vi "Process.vi"(8 "error in":errorcluster, 11 "Inst.RP100":refnum<class "Inst.RP100.lvclass">) -> (0 "error out":errorcluster, 3 "Inst.RP100 out":refnum<class "Inst.RP100.lvclass">)   [LabVIEW 2019, in "Inst.RP100.lvlib" / "Inst.RP100.lvclass"]
doc: "---------------------------------------------------------------\nJKI State Machine Objects™\nhttp://jki.net/state-machine-objects/\nCopyright (C) 2005-2015, JKI <info@jki.net>\nALL RIGHTS RESERVED"
uses:
  Inst.RP100.lvclass
  <userlib>/LevyLab/Instrument Framework/Instrument/Instrument.lvclass
  <userlib>/LevyLab/RemoteControl/RemoteControl/Typedefs/Message--Cluster.ctl
  <userlib>/LevyLab/RemoteControl/RemoteControl/RemoteControl.lvclass
  Typedefs/PrivateEvents--Inst.RP100.MessageToProcess.ctl
  C:/Program Files (x86)/National Instruments/LabVIEW 2019/user.lib/LevyLab/Instrument Framework/Instrument Types/Strain/Instrument.Strain.lvclass
  C:/Program Files (x86)/National Instruments/LabVIEW 2019/user.lib/LevyLab/Instrument Framework/Instrument/Instrument.lvclass
  C:/Program Files (x86)/National Instruments/LabVIEW 2019/vi.lib/JKI/JKI SMO/SMO/SMO.lvclass
  <userlib>/LevyLab/Debug/Debug.lvlib
  <vilib>/JKI/JKI SMO/SMO/SMO.lvclass
  <userlib>/LevyLab/Instrument Framework/Instrument Types/Strain/Instrument.Strain.lvclass
panel:
  out "Status":string
  out "State History":string
  # "Inst.RP100"
  # "Inst.RP100"
  # "For instructions on how to use the JKI State Machine Objects, examples and video tutorials, visit:\nhttp://jki.net/state-machine-objects/\n\nJKI State Machine Objects™\nhttp://jki.net/state-machine-objects/\nCopyright (C) 2005-2015, JKI <info@jki.net>\nALL RIGHTS RESERVED"
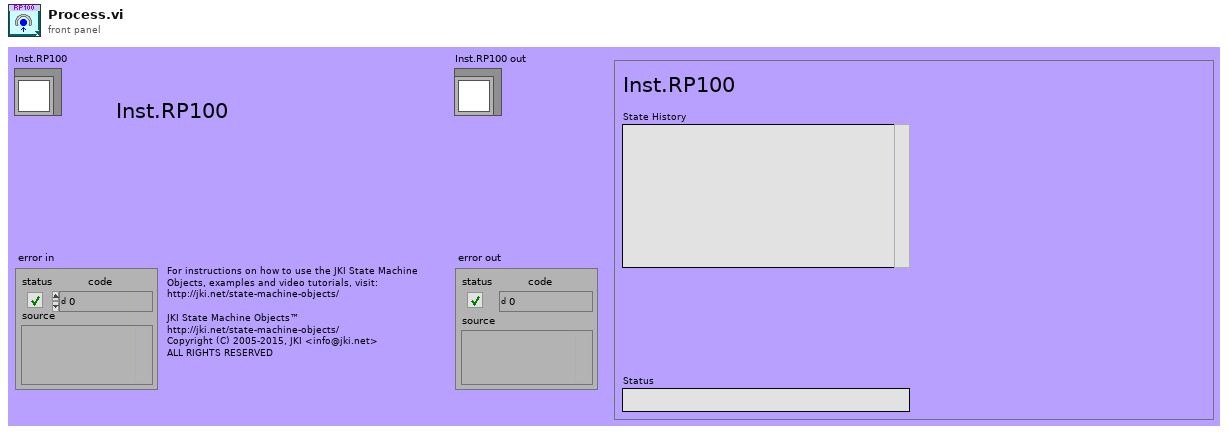
[diagram p1: front panel]
types:
  T1 = enum32{"invalid app kind", "Development System", "Run Time System", "Student Edition", "Embedded LabVIEW", "Evaluation", "Custom"}
  T2 = enum32{"Invalid", "Standard", "Closed", "Hidden", "Minimized", "Maximized"}
  T3 = typedef "RemoteControl.lvlib/RemoteControl.lvclass/Message--Cluster.ctl" = cluster{"Command":string, "Data":variant, "ID":string, "error":errorcluster}
  T4 = typedef "Inst.RP100.lvlib/Inst.RP100.lvclass/PrivateEvents--Inst.RP100.MessageToProcess.ctl" = cluster{"Message":T3}
  T5 = cluster{"Core":cluster{"Current VI Reference":refnum<vi>, "Close Panel on Exit?":bool, "Last Error":cluster{"error":errorcluster, "previous state":string, "remaining states":string}, "Shutdown?":bool}, "SMO":refnum<class "Inst.RP100.lvclass">, "Running Step":i32, "sequence":string[], "MessageToProcess":T4}
  T6 = cluster{"Current VI Reference":refnum<vi>, "Close Panel on Exit?":bool, "Last Error":cluster{"error":errorcluster, "previous state":string, "remaining states":string}, "Shutdown?":bool}
  T7 = typedef "Debug.lvlib/Attribute.Debug.lvclass/DebugBehavior.ctl" = enum16{"Normal", "Debug"}
  T8 = typedef "SMO.lvclass/Protected Events.ctl" = cluster{"StopProcesses":refnum<user-event>, "AbortProcesses":refnum<user-event>, "Config Changed":refnum<user-event>, "Dependency":refnum<user-event>}
  T9 = typedef "Inst.RP100.lvlib/Inst.RP100.lvclass/Inst.RP100.getAll--Cluster.ctl" = cluster{"OutputStateCh1":string, "OutputStateCh2":string, "LevelCh1":dbl, "LevelCh2":dbl, "SlewCh1":dbl, "SlewCh2":dbl, "MeasuredVCh1":dbl, "MeasuredVCh2":dbl, "MeasuredICh1":dbl, "MeasuredICh2":dbl}
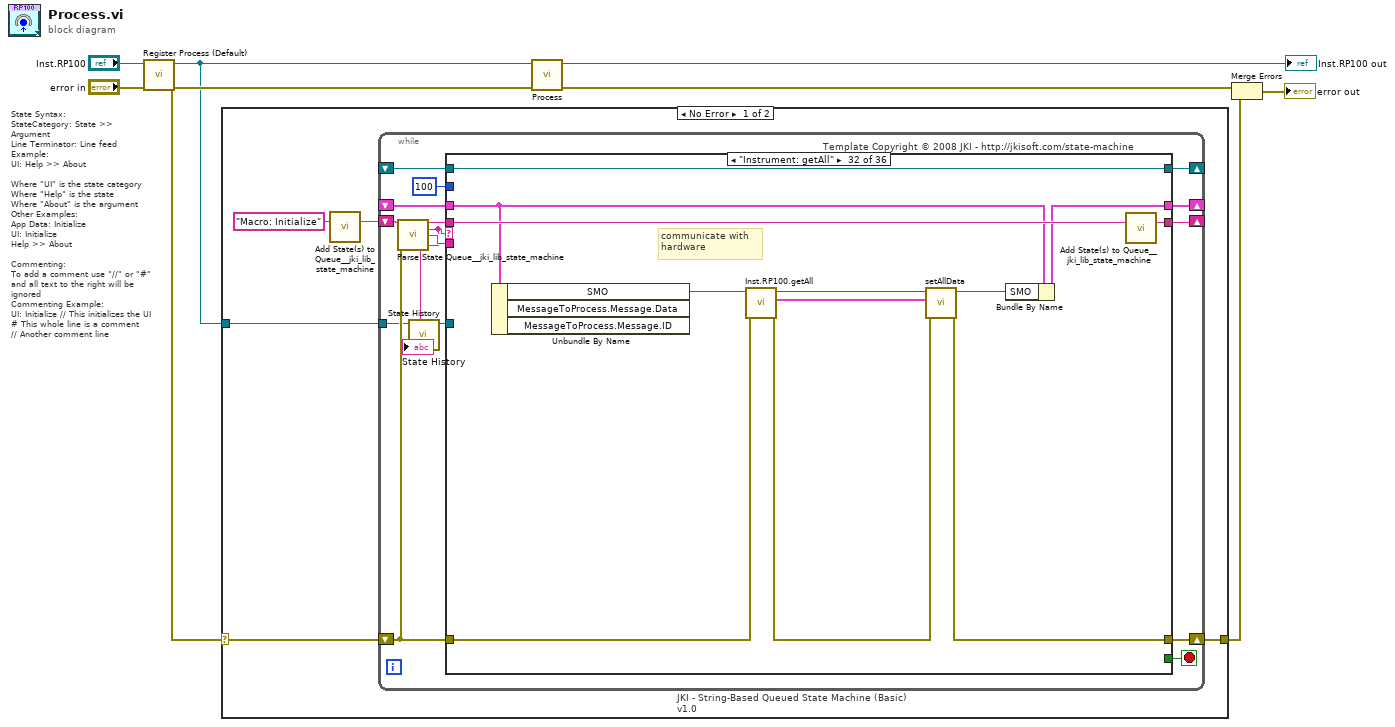
[diagram p0: block diagram]
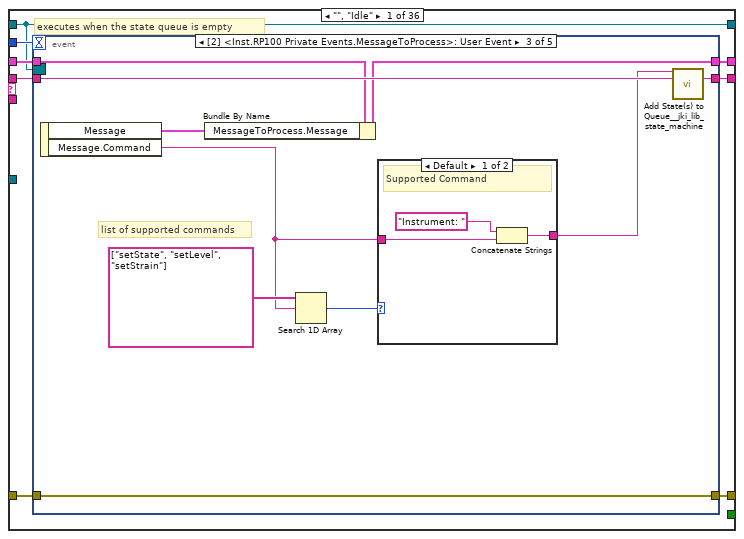
[diagram p2: hidden frame]
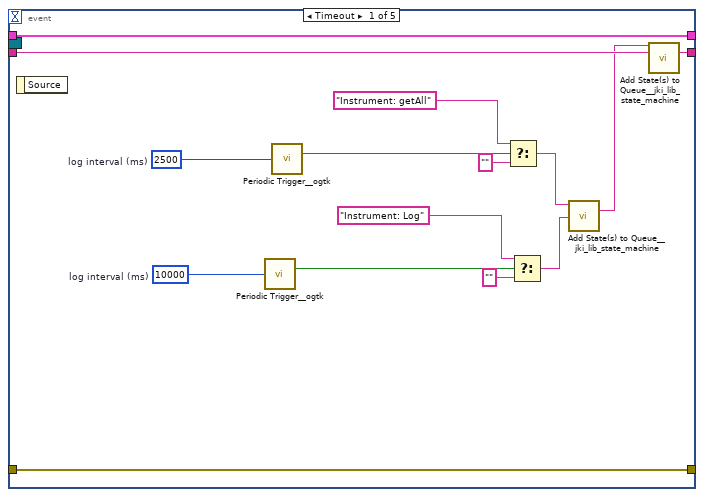
[diagram p3: hidden frame]
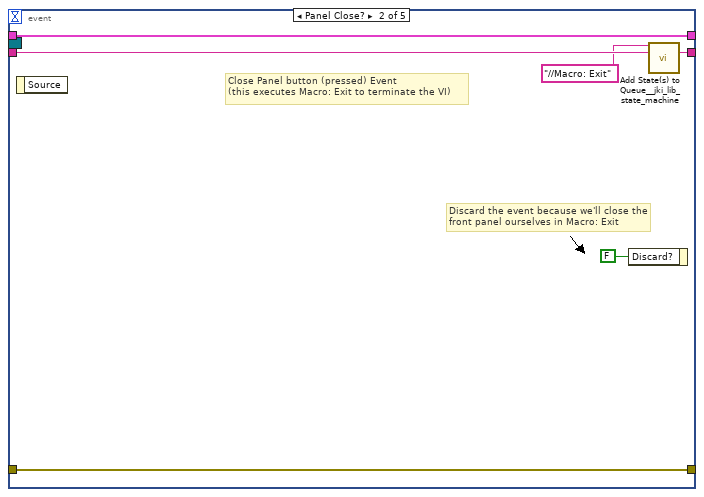
[diagram p4: hidden frame]
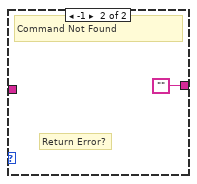
[diagram p5: hidden frame]
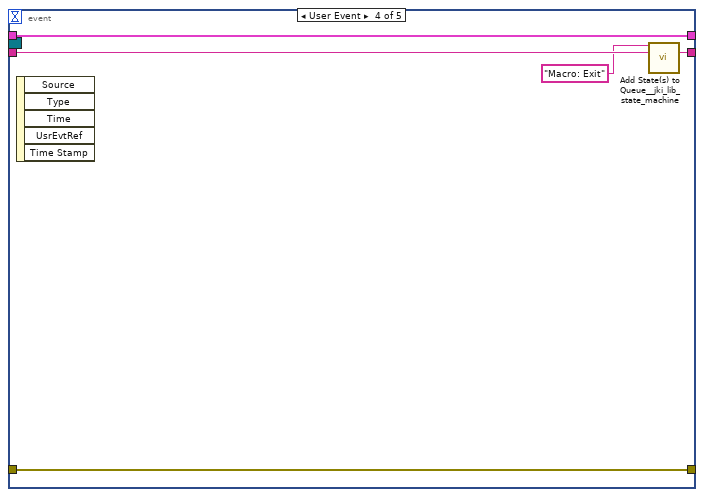
[diagram p6: hidden frame]
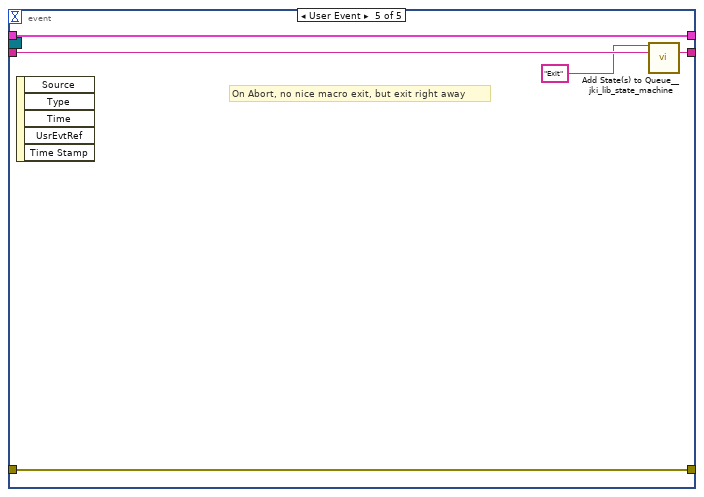
[diagram p7: hidden frame]
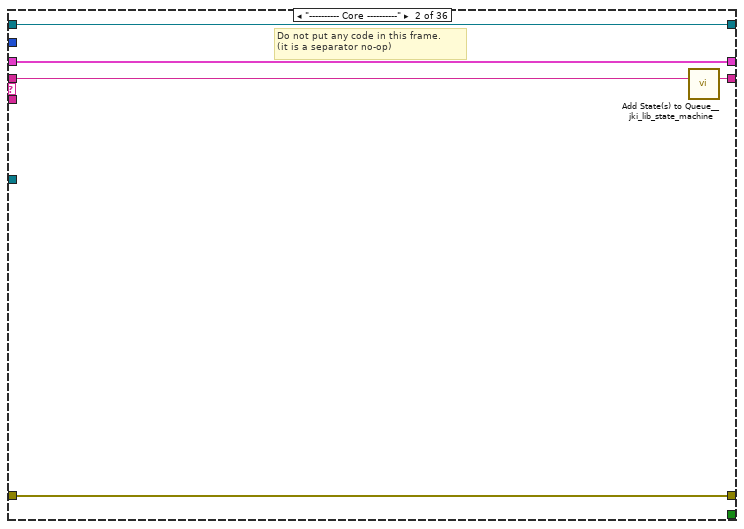
[diagram p8: hidden frame]
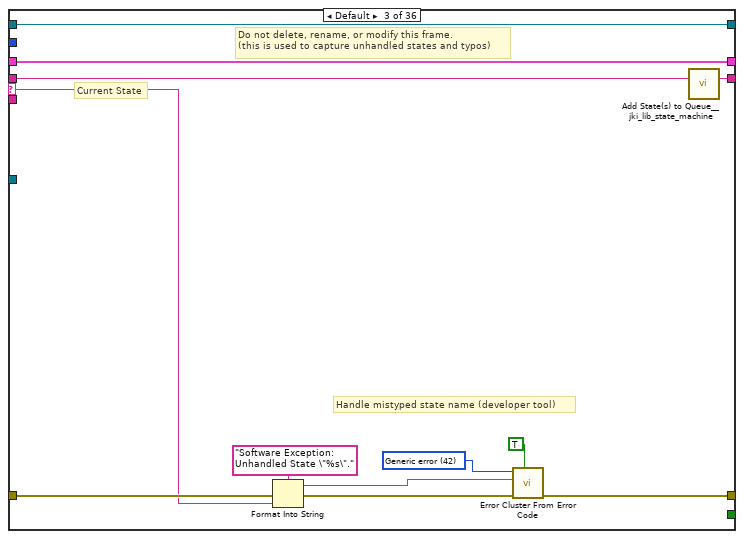
[diagram p9: hidden frame]
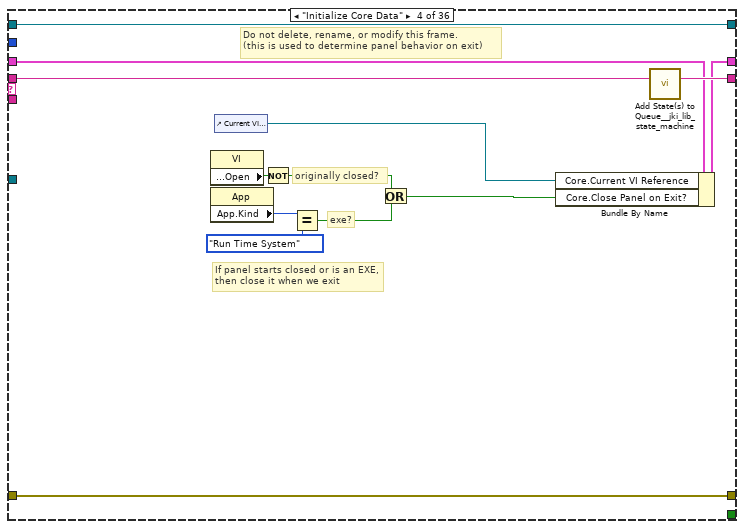
[diagram p10: hidden frame]
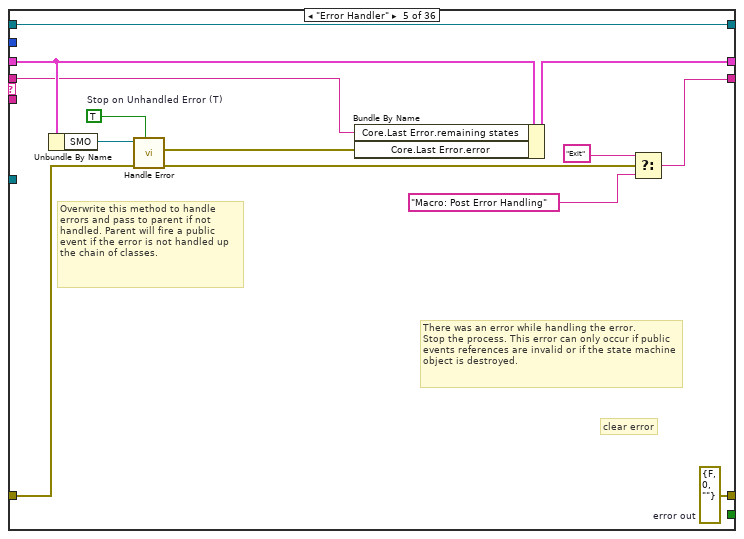
[diagram p11: hidden frame]
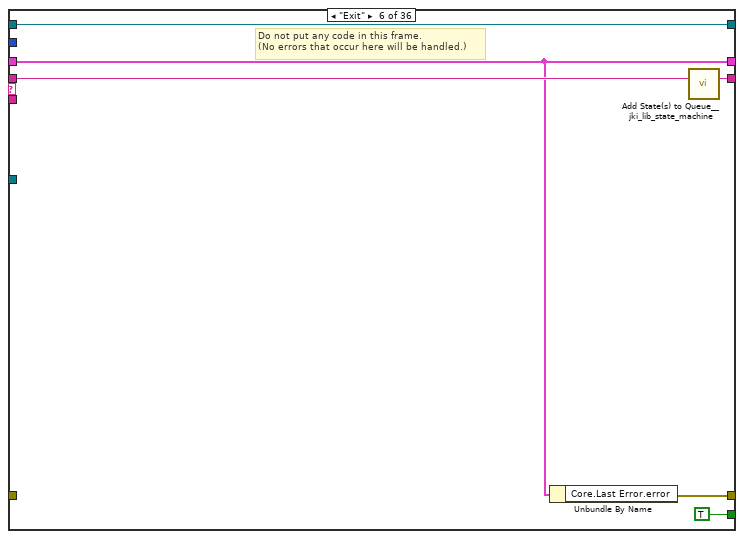
[diagram p12: hidden frame]
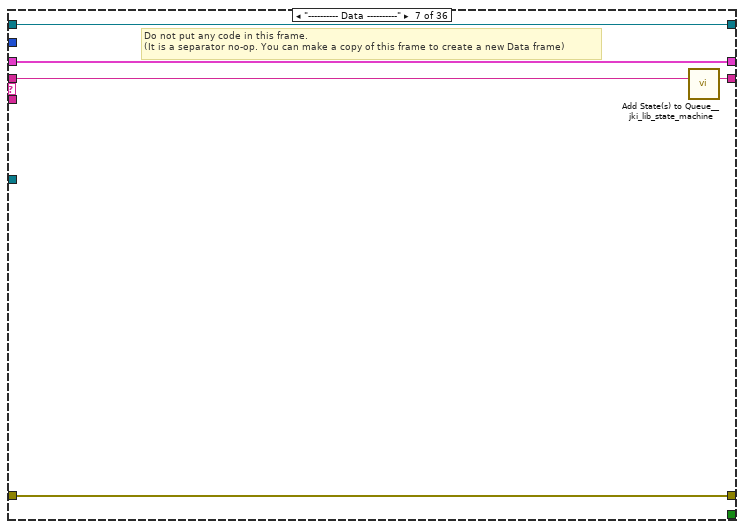
[diagram p13: hidden frame]
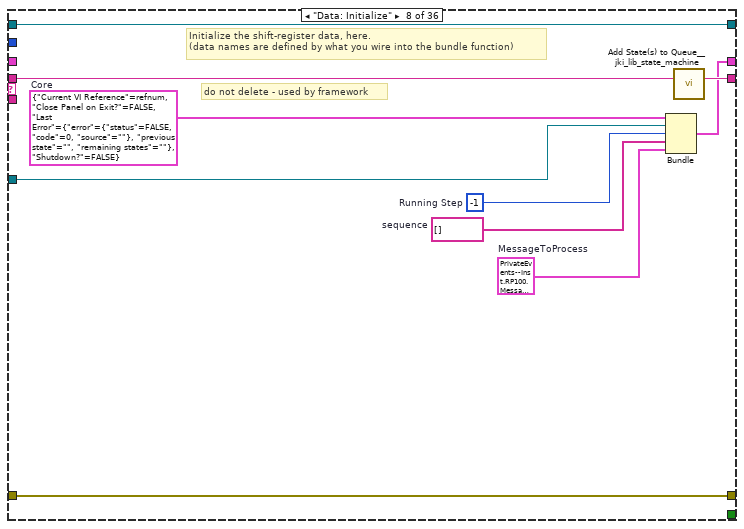
[diagram p14: hidden frame]
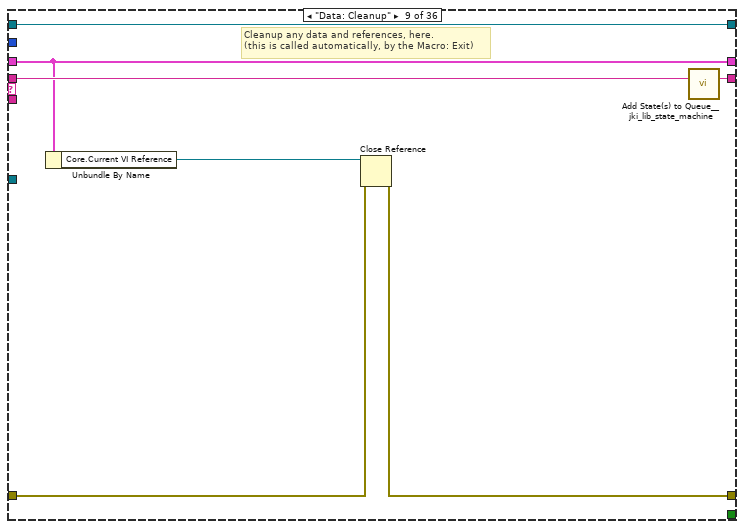
[diagram p15: hidden frame]
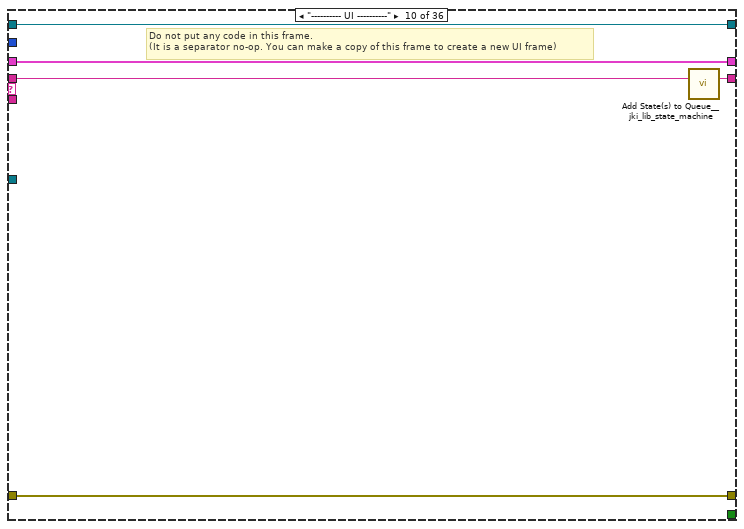
[diagram p16: hidden frame]
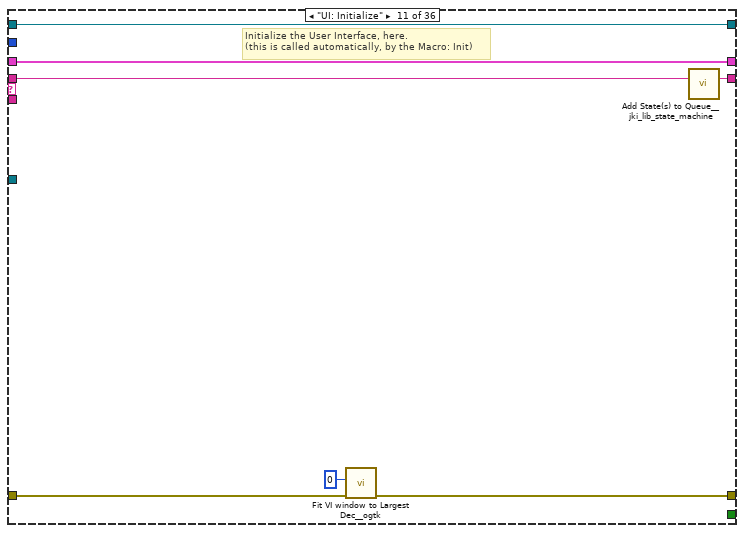
[diagram p17: hidden frame]
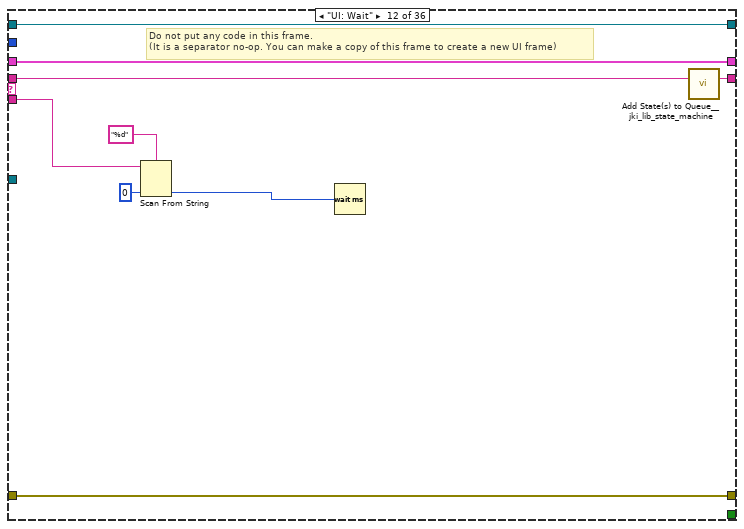
[diagram p18: hidden frame]
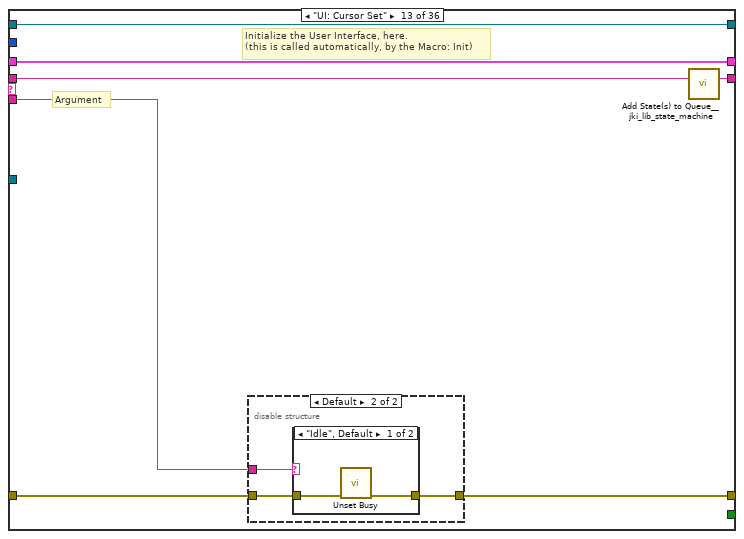
[diagram p19: hidden frame]
diagram:
  # "State Syntax:\nStateCategory: State >> Argument\nLine Terminator: Line feed\nExample:\nUI: Help >> About\n\nWhere \"UI\" is the state category\nWhere \"Help\" is the state\nWhere \"About\" is the argument\nOther Examples:\nApp Data: Initialize\nUI: Initialize\nHelp >> About\n\nCommenting:\nTo add a comment use \"//\" or \"#\" and all text to the right will be ignored\nCommenting Example:\nUI: Initialize // This initializes the UI\n# This whole line is a comment\n// Another comment line"
  n1 = call <vilib>:"Register Process (Default).vi"("error in (no error)"="error in", "SMO"="Inst.RP100") -> ("error out"=w5:errorcluster, "SelfRef"=w4:refnum<class "Inst.RP100.lvclass">)  [unwired: 8 in]
  n2 = case shown="No Error" w5 {
    selector: w5 -> [w10 w459]
    tunnel: w4 -> [w11 _]
    tunnel: [w9 w459] -> w1
    frame No Error {
      n3 = call <vilib>:"Add State(s) to Queue__jki_lib_state_machine.vi"("State(s) in (\"\")"="Macro: Initialize") -> ("States Out"=w13:string)  [unwired: 14 in]
      n4 = while "JKI - String-Based Queued State Machine (Basic) v1.0" {
        shift-right: [w23] -> _
        shift-left: _ -> [w22]
        shift-right: [w26] -> w9
        shift-left: w10 -> [w20]
        shift-right: [w25] -> _
        shift-left: w13 -> [w27]
        tunnel: w11 -> [w14]
        shift-right: [w19] -> _
        shift-left: _ -> [w18]
        stop <- w24 stop-if-true
        # "Template Copyright © 2008 JKI - http://jkisoft.com/state-machine"
        n5 = call <vilib>:"Parse State Queue__jki_lib_state_machine.vi"("State Queue"=w27, "Error In (no error)"=w20) -> ("Remaining States"=w29:string, "Current State"=w17:string, "Arguments"=w28:string)  [unwired: 11 in]
        n6 = call <userlib>:"State History.vi"("Current State"=w17, "SMO"=w14) -> ("SMO"=w15:refnum<class "Inst.RP100.lvclass">, "History"=→"State History":string)  [unwired: 8 in]
        n7 = case shown="\"Instrument: getAll\"" w17 {
          selector: w17 -> [_ _ w89 _ _ _ _ _ _ _ _ _ _ _ _ _ _ _ _ _ _ _ _ _ _ _ _ _ _ _ _ _ _ _ _ _]
          tunnel: w29 -> [w37 w87 w93 w112 w117 w131 w136 w146 w153 w158 w165 w174 w181 w197 w229 w238 w253 w270 w291 w308 w313 w324 w329 w342 w348 w355 w364 w373 w383 w393 w403 w415 w428 w433 w439 w458]
          tunnel: w28 -> [_ _ _ _ _ _ _ _ _ _ _ w166 w175 w191 _ _ _ _ _ _ _ _ _ _ _ _ _ _ _ _ _ _ _ _ w434 w442]
          tunnel: w22 -> [w35 w84 w91 w103 w121 w127 w133 _ w147 w155 w163 w171 w179 w193 w226 w235 w242 w260 w281 w292 w310 w321 w326 w335 w346 w350 w360 w369 w379 w389 w399 w411 w424 w429 w435 w448]
          tunnel: [w34 w85 w95 w109 w122 w126 w134 w138 w149 w156 w160 w172 w176 w194 w227 w230 w240 w268 w289 w295 w311 w315 w327 w338 w344 w352 w357 w366 w375 w385 w395 w404 w418 w430 w436 w450] -> w26
          tunnel: w20 -> [w33 w85 w94 w109 w123 _ w134 w138 w150 w156 w159 w172 w177 w195 w227 w230 w239 w268 w289 w295 w311 w316 w327 w332 w344 w352 w356 w365 w376 w386 w396 w409 w419 w430 w436 w444]
          tunnel: [w36 w86 w92 w111 w113 w130 w135 w145 w152 w157 w164 w173 w180 w196 w228 w237 w252 w269 w290 w307 w312 w323 w328 w341 w347 w354 w363 w372 w382 w392 w402 w414 w427 w432 w438 w457] -> w25
          tunnel: [_ _ _ _ _ TRUE _ _ _ _ _ _ _ _ _ _ _ _ _ _ _ _ _ _ _ _ _ _ _ _ _ _ _ _ _ _] -> w24
          tunnel: [w32 w84 w91 w110 w120 w127 w133 w144 w147 w155 w163 w171 w179 w193 w226 w235 w243 w261 w282 w293 w310 w321 w326 w335 w346 w351 w361 w370 w380 w390 w400 w412 w425 w429 w435 w447] -> w23
          tunnel: 100 ("Timeout") -> [w31 _ _ _ _ _ _ _ _ _ _ _ _ _ _ _ _ _ _ _ _ _ _ _ _ _ _ _ _ _ _ _ _ _ _ _]
          tunnel: w15 -> [_ _ _ _ _ _ _ w139 _ _ _ _ _ _ _ _ _ _ _ _ _ _ _ _ _ _ _ _ _ _ _ _ _ _ _ _]
          tunnel: [w30 w83 w88 w100 w125 w128 w132 w143 w148 w154 w162 w170 w178 w190 w225 w236 w251 w267 w288 w302 w309 w322 w325 w340 w345 w353 w362 w371 w381 w391 w401 w413 w426 w431 w437 w456] -> w19
          tunnel: w18 -> [w30 w83 w88 w100 w125 w128 w132 w143 w148 w154 w162 w170 w178 w190 w225 w236 w251 w267 w288 w302 w309 w322 w325 _ w345 w353 w362 w371 w381 w391 w401 w413 w426 w431 w437 w456]
          frame "", "Idle" {
            # "executes when the state queue is empty"
            n8 = event shown="[2] <Inst.RP100 Private Events.MessageToProcess>: User Event" {
              selector: w30 -> [_ _ _ _ _]
              dyn-events: _ -> [_ _ _ _ _]
              timeout: w31 -> [_ _ _ _ _]
              tunnel: w37 -> [w52 w58 w68 w77 w82]
              tunnel: [w51 w57 w67 w76 w81] -> w36
              tunnel: w35 -> [w49 w55 w60 w74 w79]
              tunnel: [w50 w56 w66 w75 w80] -> w34
              tunnel: w33 -> [w50 w56 w66 w75 w80]
              tunnel: [w49 w55 w61 w74 w79] -> w32
              event Timeout {
                w42 = u32 10000  # log interval (ms)
                w46 = u32 2500  # log interval (ms)
                n9 = event-data() -> ()  [unwired: 1 in, 1 out]
                n10 = call <userlib>:"Periodic Trigger__ogtk.vi"("time (ms)"=w42) -> ("Triggered"=w41:bool)  [unwired: 12 in, 2 out]
                n11 = call <userlib>:"Periodic Trigger__ogtk.vi"("time (ms)"=w46) -> ("Triggered"=w48:bool)  [unwired: 12 in, 2 out]
                n12 = Select(t="Instrument: getAll", s=w48, f="") -> (s? t:f=w39:string)
                n13 = Select(t="Instrument: Log", s=w41, f="") -> (s? t:f=w40:string)
                n14 = call <vilib>:"Add State(s) to Queue__jki_lib_state_machine.vi"("State(s) in Front (\"\")"=w39, "State(s) at Back (\"\")"=w40) -> ("States Out"=w38:string)  [unwired: 13 in]
                n15 = call <vilib>:"Add State(s) to Queue__jki_lib_state_machine.vi"("State(s) in Front (\"\")"=w38, "State(s) in (\"\")"=w52) -> ("States Out"=w51:string)  [unwired: 13 in]
              }
              event Panel Close? {
                # "Discard the event because we'll close the front panel ourselves in Macro: Exit"
                # "Close Panel button (pressed) Event\n(this executes Macro: Exit to terminate the VI)"
                n16 = event-data() -> ()  [unwired: 1 in, 1 out]
                n17 = event-data("Discard?"=FALSE) -> ()  [unwired: 1 in, 1 out]
                n18 = call <vilib>:"Add State(s) to Queue__jki_lib_state_machine.vi"("State(s) in Front (\"\")"="//Macro: Exit", "State(s) in (\"\")"=w58) -> ("States Out"=w57:string)  [unwired: 13 in]
              }
              event User Event {
                # "list of supported commands"
                n19 = event-data() -> ("Message"=w59:T3, "Message.Command"=w62:string)  [unwired: 1 in]
                n20 = Bundle By Name(cluster=w60, "MessageToProcess.Message"=w59) -> (w61:T5)
                n21 = Search 1D Array(1D array=string[] ["setState", "setLevel", "setStrain"], element=w62) -> (index of element=w65:i32)  [unwired: 1 in]
                n22 = case shown="Default" w65 {
                  tunnel: [w71 "" ("Empty String Constant")] -> w63
                  tunnel: w62 -> [w70 _]
                  frame Default {
                    # "Supported Command"
                    n23 = Concatenate Strings("Instrument: ", w70) -> (w71:string)
                  }
                  frame -1 {
                    # "Return Error?"
                    # "Command Not Found"
                  }
                }
                n24 = call <vilib>:"Add State(s) to Queue__jki_lib_state_machine.vi"("State(s) in Front (\"\")"=w63, "State(s) in (\"\")"=w68) -> ("States Out"=w67:string)  [unwired: 13 in]
              }
              event User Event {
                n25 = event-data() -> ()  [unwired: 1 in, 5 out]
                n26 = call <vilib>:"Add State(s) to Queue__jki_lib_state_machine.vi"("State(s) in Front (\"\")"="Macro: Exit", "State(s) in (\"\")"=w77) -> ("States Out"=w76:string)  [unwired: 13 in]
              }
              event User Event {
                # "On Abort, no nice macro exit, but exit right away"
                n27 = event-data() -> ()  [unwired: 1 in, 5 out]
                n28 = call <vilib>:"Add State(s) to Queue__jki_lib_state_machine.vi"("State(s) in Front (\"\")"="Exit", "State(s) in (\"\")"=w82) -> ("States Out"=w81:string)  [unwired: 13 in]
              }
            }
          }
          frame "---------- Core ----------" {
            # "Do not put any code in this frame.\n(it is a separator no-op)"
            n29 = call <vilib>:"Add State(s) to Queue__jki_lib_state_machine.vi"("State(s) in (\"\")"=w87) -> ("States Out"=w86:string)  [unwired: 14 in]
          }
          frame Default {
            w98 = 42 items=["No error", "Argument error", "Memory is full", "Out of zone", "End of file", "File already open", "Generic file I/O error", "File not found", "File permission error", "Disk is full", "Duplicate path", "Too many files open", "System feature not enabled", "Resource file not found", "Cannot add resource", "Resource not found", "Image not found", "Image memory error", "Pen does not exist", "Config type invalid", "Config token not found", "Config parse error", "Config memory error", "Bad external code format", "Bad external code offset", "External code not present", "Null window", "Destroy window error", "Null menu", "Print aborted", "Bad print record", "Print driver error", "Windows error during printing", "Memory error during printing", "Print dialog error", "Generic print error", "Invalid device refnum", "Device not found", "Device parameter error", "Device unit error", "Cannot open device", "Device call aborted", "Generic error", "Cancelled by user", "Object ID too low", "Object ID too high", "Object not in heap", "Unknown heap", "Unknown object (invalid DefProc)", "Unknown object (DefProc not in table)", "Message out of range", "Invalid (null) method", "Unknown message", "Manager call not supported", "Bad address", "Network operation in progress", "Network operation timed out", "Connection is busy", "Network attribute not supported", "Network error", "Address in use", "System out of memory", "Connection aborted", "Connection refused", "Not connected", "Already connected", "Connection closed", "Initialization error (interapplication manager)", "Bad occurrence", "Wait on unbound occurrence handler", "Occurrence queue overflow", "Datalog type conflict", "Unused", "Unrecognized type (interapplication manager)", "Memory corrupt", "Failed to make temporary DLL", "Old CIN version", "Drag socket not found", "Failed to load drop-object", "Failed to register OLE object", "Failed to release OLE object", "Format specifier type mismatch", "Unknown format specifier", "Too few format specifiers", "Too many format specifiers", "Scan failed", "Newer CIN version", "Error converting to variant", "Runtime menu error", "Password tampered", "Variant attribute not found", "Incompatible variant data type", "Event data is not available", "Event Store is not present", "Occurrence is not found", "Event Queue is not created", "Event info is not available", "Refnum passed is NULL", "Error retrieving Class GUID", "Error retrieving CoClass GUID", "Error retrieving TypeLib GUID.", "Bad built application magic bytes.", "Specific driver is different from the specific driver associated with the Logical Name.", "There is no session opened to the class driver.", "Max Error", "MAX - Error with config objects", "MAX - Error loading configuration", "MAX - Group not supported"]
            # "Current State"
            # "Do not delete, rename, or modify this frame.\n(this is used to capture unhandled states and typos)"
            # "Handle mistyped state name (developer tool)"
            n30 = Format Into String(format string="Software Exception: Unhandled State \"%s\"." ("message"), error in=w94, w89) -> (resulting string=w97:string, error out=w96:errorcluster)  [unwired: 1 in]
            n31 = call <vilib>:"Error Cluster From Error Code.vi"("show call chain? (False)"=TRUE, "error in (no error)"=w96, "error message (\"\")"=w97, "error code (0)"=w98) -> ("error out"=w95:errorcluster)  [unwired: 5 in]
            n32 = call <vilib>:"Add State(s) to Queue__jki_lib_state_machine.vi"("State(s) in (\"\")"=w93) -> ("States Out"=w92:string)  [unwired: 14 in]
          }
          frame "Initialize Core Data" {
            # "Do not delete, rename, or modify this frame.\n(this is used to determine panel behavior on exit)"
            # "originally closed?"
            # "exe?"
            # "If panel starts closed or is an EXE, then close it when we exit"
            n33 = property class="VI"() -> ("Front Panel.Open"=w108:bool)  [unwired: 2 in, 2 out]
            n34 = property class="App"() -> ("App.Kind"=w107:T1)  [unwired: 2 in, 2 out]
            n35 = control-ref of="Current VI Reference"() -> (w101:refnum<vi>)
            n36 = Not(x=w108) -> (.not. x?=w105:bool)
            n37 = Equal?(x=w107, y=T1."Run Time System" ("Application:Kind")) -> (x = y?=w104:bool)
            n38 = Or(x=w105, y=w104) -> (x .or. y?=w102:bool)
            n39 = Bundle By Name(cluster=w103, "Core.Current VI Reference"=w101, "Core.Close Panel on Exit?"=w102) -> (w110:T5)
            n40 = call <vilib>:"Add State(s) to Queue__jki_lib_state_machine.vi"("State(s) in (\"\")"=w112) -> ("States Out"=w111:string)  [unwired: 14 in]
          }
          frame "Error Handler" {
            w118 = TRUE  # Stop on Unhandled Error (T)
            w122 = errorcluster {"status"=FALSE, "code"=0, "source"=""}  # error out
            # "clear error"
            # "There was an error while handling the error.\nStop the process. This error can only occur if public events references are invalid or if the state machine object is destroyed."
            # "Overwrite this method to handle errors and pass to parent if not handled. Parent will fire a public event if the error is not handled up the chain of classes."
            n41 = Unbundle By Name(w121) -> ("SMO"=w124:refnum<class "Inst.RP100.lvclass">)
            n42 = call-dynamic "Handle Error.vi"("Stop on Unhandled Error (T)"=w118, "error in"=w123, "SMO"=w124) -> ("handling error"=w114:errorcluster, "Unhandled error"=w119:errorcluster)  [unwired: 6 in, 1 out]
            n43 = Bundle By Name(cluster=w121, "Core.Last Error.remaining states"=w117, "Core.Last Error.error"=w119) -> (w120:T5)
            n44 = Select(t="Exit", s=w114, f="Macro: Post Error Handling") -> (s? t:f=w113:string)
          }
          frame "Exit" {
            # "Do not put any code in this frame.\n(No errors that occur here will be handled.)"
            n45 = Unbundle By Name(w127) -> ("Core.Last Error.error"=w126:errorcluster)
            n46 = call <vilib>:"Add State(s) to Queue__jki_lib_state_machine.vi"("State(s) in (\"\")"=w131) -> ("States Out"=w130:string)  [unwired: 14 in]
          }
          frame "---------- Data ----------" {
            # "Do not put any code in this frame.\n(It is a separator no-op. You can make a copy of this frame to create a new Data frame)"
            n47 = call <vilib>:"Add State(s) to Queue__jki_lib_state_machine.vi"("State(s) in (\"\")"=w136) -> ("States Out"=w135:string)  [unwired: 14 in]
          }
          frame "Data: Initialize" {
            w137 = T4 {"Message"={"Command"="", "Data"=variant(string ""), "ID"="", "error"={"status"=FALSE, "code"=0, "source"=""}}}  # MessageToProcess
            w140 = string[] []  # sequence
            w141 = -1  # Running Step
            w142 = T6 {"Current VI Reference"=refnum, "Close Panel on Exit?"=FALSE, "Last Error"={"error"={"status"=FALSE, "code"=0, "source"=""}, "previous state"="", "remaining states"=""}, "Shutdown?"=FALSE}  # Core
            # "do not delete - used by framework"
            # "Initialize the shift-register data, here.\n(data names are defined by what you wire into the bundle function)"
            n48 = Bundle("Core"=w142, "SMO"=w139, "Running Step"=w141, "sequence"=w140, "MessageToProcess"=w137) -> (w144:T5)  [unwired: 1 in]
            n49 = call <vilib>:"Add State(s) to Queue__jki_lib_state_machine.vi"("State(s) in (\"\")"=w146) -> ("States Out"=w145:string)  [unwired: 14 in]
          }
          frame "Data: Cleanup" {
            # "Cleanup any data and references, here.\n(this is called automatically, by the Macro: Exit)"
            n50 = Unbundle By Name(w147) -> ("Core.Current VI Reference"=w151:refnum<vi>)
            n51 = Close Reference(reference=w151, error in (no error)=w150) -> (error out=w149:errorcluster)
            n52 = call <vilib>:"Add State(s) to Queue__jki_lib_state_machine.vi"("State(s) in (\"\")"=w153) -> ("States Out"=w152:string)  [unwired: 14 in]
          }
          frame "---------- UI ----------" {
            # "Do not put any code in this frame.\n(It is a separator no-op. You can make a copy of this frame to create a new UI frame)"
            n53 = call <vilib>:"Add State(s) to Queue__jki_lib_state_machine.vi"("State(s) in (\"\")"=w158) -> ("States Out"=w157:string)  [unwired: 14 in]
          }
          frame "UI: Initialize" {
            # "Initialize the User Interface, here.\n(this is called automatically, by the Macro: Init)"
            n54 = call <userlib>:"Fit VI window to Largest Dec__ogtk.vi"("error in (no error)"=w159, "border spacing (2 px)"=0) -> ("error out"=w160:errorcluster)  [unwired: 4 in, 1 out]
            n55 = call <vilib>:"Add State(s) to Queue__jki_lib_state_machine.vi"("State(s) in (\"\")"=w165) -> ("States Out"=w164:string)  [unwired: 14 in]
          }
          frame "UI: Wait" {
            # "Do not put any code in this frame.\n(It is a separator no-op. You can make a copy of this frame to create a new UI frame)"
            n56 = Scan From String(format string="%d", input string=w166, default 1=u32 0 ("default value 1")) -> (output 1=w167:u32)  [unwired: 2 in, 3 out]
            n57 = Wait (ms)(milliseconds to wait=w167) -> ()  [unwired: 1 out]
            n58 = call <vilib>:"Add State(s) to Queue__jki_lib_state_machine.vi"("State(s) in (\"\")"=w174) -> ("States Out"=w173:string)  [unwired: 14 in]
          }
          frame "UI: Cursor Set" {
            # "Argument"
            # "Initialize the User Interface, here.\n(this is called automatically, by the Macro: Init)"
            n59 = disable-structure shown="Default" {
              disable-tunnel: w177 -> [w182 w185]
              disable-tunnel: [w182 w184] -> w176
              disable-tunnel: w175 -> [_ w183]
              frame condition #0 {
              }
              frame condition #1 (active) {
                n60 = case shown="\"Idle\", Default" w183 {
                  tunnel: w185 -> [w187 w189]
                  tunnel: [w186 w188] -> w184
                  frame "Idle", Default {
                    n61 = call <vilib>:"Unset Busy.vi"("error in (no error)"=w187) -> ("error out"=w186:errorcluster)  [unwired: 10 in]
                  }
                  frame "Busy" {
                    n62 = call <vilib>:"Set Busy.vi"("error in (no error)"=w189) -> ("error out"=w188:errorcluster)  [unwired: 9 in, 1 out]
                  }
                }
              }
            }
            n63 = call <vilib>:"Add State(s) to Queue__jki_lib_state_machine.vi"("State(s) in (\"\")"=w181) -> ("States Out"=w180:string)  [unwired: 14 in]
          }
          frame "UI: Front Panel State" {
            # "Argument"
            # "Set Front Panel Open or Closed\n(Usage: \"UI: Front Panel State >> Open|Close\")"
            n64 = Unbundle By Name(w193) -> ("Core.Current VI Reference"=w192:refnum<vi>)
            n65 = disable-structure shown="Default" {
              disable-tunnel: w195 -> [w201 w224]
              disable-tunnel: [w200 w224] -> w194
              disable-tunnel: w192 -> [w199 _]
              disable-tunnel: w191 -> [w198 _]
              frame condition #0 (active) {
                n66 = case shown="\"Close\"" w198 {
                  tunnel: w201 -> [w205 w218]
                  tunnel: [w207 w219] -> w200
                  tunnel: w199 -> [w206 w216]
                  frame "Open", Default {
                    n67 = property class="VI"(reference=w206, error in=w205) -> (reference out=w203:refnum<vi>, error out=w204:errorcluster, "FP.State"=w202:T2)
                    n68 = case shown="\"Closed\"" w202 {
                      tunnel: [w210 w213] -> w207
                      tunnel: w204 -> [w209 w213]
                      tunnel: w203 -> [w208 _]
                      frame "Closed" {
                        n69 = invoke class="VI" method="FP.Open"(reference=w208, error in=w209, "Activate"=TRUE, "State"=T2."Standard") -> (error out=w210:errorcluster)  [unwired: 1 in, 4 out]
                      }
                      frame Default {
                      }
                    }
                  }
                  frame "Close" {
                    n70 = property class="VI"(reference=w216, error in=w218) -> (reference out=w215:refnum<vi>, error out=w217:errorcluster, "FP.State"=w214:T2)
                    n71 = case shown="Default" w214 {
                      tunnel: [w220 w223] -> w219
                      tunnel: w217 -> [w220 w222]
                      tunnel: w215 -> [_ w221]
                      frame "Invalid", "Closed" {
                      }
                      frame Default {
                        n72 = invoke class="VI" method="FP.Close"(reference=w221, error in=w222) -> (error out=w223:errorcluster)  [unwired: 1 in, 2 out]
                      }
                    }
                  }
                }
              }
              frame condition #1 {
              }
            }
            n73 = call <vilib>:"Add State(s) to Queue__jki_lib_state_machine.vi"("State(s) in (\"\")"=w197) -> ("States Out"=w196:string)  [unwired: 14 in]
          }
          frame "---------- Macro ----------" {
            # "Do not put any code in this frame.\n(It is a separator no-op. You can make a copy of this frame to create a new Macro frame)"
            n74 = call <vilib>:"Add State(s) to Queue__jki_lib_state_machine.vi"("State(s) in (\"\")"=w229) -> ("States Out"=w228:string)  [unwired: 14 in]
          }
          frame "Macro: Initialize" {
            # "Initialization Macro\n(This is called once, when the VI starts)"
            n75 = call <vilib>:"Add State(s) to Queue__jki_lib_state_machine.vi"("State(s) in Front (\"\")"="Data: Initialize\nInitialize Core Data\nEvents: Register", "State(s) in (\"\")"="Process: Sync", "State(s) at Back (\"\")"="UI: Initialize\nUI: Front Panel State >> Close\nMacro: Debug\nInstrument: Open Hardware\nInstrument: getAll") -> ("States Out"=w233:string)  [unwired: 12 in]
            n76 = call <vilib>:"Add State(s) to Queue__jki_lib_state_machine.vi"("State(s) in Front (\"\")"=w233, "State(s) in (\"\")"=w238) -> ("States Out"=w237:string)  [unwired: 13 in]
          }
          frame "Macro: Debug" {
            # "exe?"
            # "If pane is an EXE, then close it when we exit"
            # "Macro: Debug\n(get debug behavior, determine UI and determine shutdown behavior)"
            n77 = Unbundle By Name(w242) -> ("Core.Close Panel on Exit?"=w245:bool, "SMO"=w250:refnum<class "Inst.RP100.lvclass">)
            n78 = property class="App"() -> ("App.Kind"=w248:T1)  [unwired: 2 in, 2 out]
            n79 = Equal?(x=w248, y=T1."Run Time System" ("Application:Kind")) -> (x = y?=w244:bool)
            n80 = call <userlib>:"Get Debug Mode.vi"("error in (no error)"=w239, "SMO"=w250) -> ("error out"=w240:errorcluster, "Behavior"=w249:T7)  [unwired: 7 in, 1 out]
            n81 = case shown="\"Debug\"" w249 {
              tunnel: [w254 w256] -> w246
              tunnel: w245 -> [w254 _]
              tunnel: w244 -> [_ w258]
              tunnel: [_ "UI: Front Panel State >> Open\nUI: Wait >> 1000"] -> w241
              frame "Normal", Default {
                # "respect core.close"
              }
              frame "Debug" {
                # "keep panel open\nunless exe"
                n82 = Or(x=w258, y=FALSE) -> (x .or. y?=w256:bool)
              }
            }
            n83 = Bundle By Name(cluster=w242, "Core.Close Panel on Exit?"=w246) -> (w243:T5)
            n84 = call <vilib>:"Add State(s) to Queue__jki_lib_state_machine.vi"("State(s) in Front (\"\")"=w241, "State(s) in (\"\")"=w253) -> ("States Out"=w252:string)  [unwired: 13 in]
          }
          frame "Macro: Post Error Handling" {
            # "Clear Last Error?"
            n85 = Unbundle By Name(w260) -> ("Core.Last Error.remaining states"=w262:string, "Core.Shutdown?"=w263:bool)
            n86 = Unbundle By Name(w260) -> ("Core.Last Error.error"=w266:errorcluster)
            n87 = case shown="False" FALSE {
              tunnel: w266 -> [w274 _]
              tunnel: [w274 _] -> w265
              frame False {
              }
              frame True {
              }
            }
            n88 = case shown="True" w263 {
              tunnel: w262 -> [w271 w273]
              tunnel: [w271 w272] -> w259
              frame False {
                # "These are the remaining states (at the moment the error occured). States can be altered according to business logic."
                # "NOT SHUTTING DOWN"
              }
              frame True {
                # "Developer can decide to alter the states but should be aware that during the shutdown process, there are certain states that must be run for the SMO to properly shut itself (and this process) down. As such, one can add states to perform additional clean-ups, but should append the remaining state to be executed."
                # "SHUTTING DOWN"
                n89 = call <vilib>:"Add State(s) to Queue__jki_lib_state_machine.vi"("State(s) in (\"\")"=w273) -> ("States Out"=w272:string)  [unwired: 14 in]
              }
            }
            n90 = Bundle By Name(cluster=w260, "Core.Last Error.error"=w265) -> (w261:T5)
            n91 = call <vilib>:"Add State(s) to Queue__jki_lib_state_machine.vi"("State(s) in Front (\"\")"=w259, "State(s) in (\"\")"=w270) -> ("States Out"=w269:string)  [unwired: 13 in]
          }
          frame "Macro: Run Sequence" {
            # "0,1,2,3,4,"
            # "5"
            # "Do not put any code in this frame.\n(It is a separator no-op. You can make a copy of this frame to create a new Macro frame)"
            n92 = Unbundle By Name(w281) -> ("sequence"=w277:string[], "Running Step"=w275:i32)
            n93 = Array Size(array=w277) -> (size(s)=w287:i32)
            n94 = Index Array(array=w277, index=w275) -> (element=w276:string)
            n95 = Greater Or Equal?(x=w287, y=w275) -> (x >= y?=w279:bool)
            n96 = Select(t=-1 ("Running Step"), s=w279, f=w275) -> (s? t:f=w286:i32)
            n97 = Bundle By Name(cluster=w281, "Running Step"=w286) -> (w282:T5)
            n98 = Select(t="Sequence: Status >> ...", s=w279, f="Idle //Check Event Structure\nMacro: Run Sequence" ("State(s) at Back (\"\")")) -> (s? t:f=w278:string)
            n99 = call <vilib>:"Add State(s) to Queue__jki_lib_state_machine.vi"("State(s) in Front (\"\")"=w276, "State(s) at Back (\"\")"=w278) -> ("States Out"=w280:string)  [unwired: 13 in]
            n100 = call <vilib>:"Add State(s) to Queue__jki_lib_state_machine.vi"("State(s) in Front (\"\")"=w280, "State(s) in (\"\")"=w291) -> ("States Out"=w290:string)  [unwired: 13 in]
          }
          frame "Macro: Exit" {
            # "Exit Macro\n(This is called once, when the VI exits)"
            n101 = Unbundle By Name(w292) -> ("Core.Close Panel on Exit?"=w306:bool)
            n102 = Bundle By Name(cluster=w292, "Core.Shutdown?"=TRUE) -> (w293:T5)
            n103 = Select(t="UI: Front Panel State >> Close", s=w306, f="" ("Empty String Constant")) -> (s? t:f=w304:string)
            n104 = call <vilib>:"Add State(s) to Queue__jki_lib_state_machine.vi"("State(s) in Front (\"\")"="Data: Cleanup\nEvents: Unregister", "State(s) in (\"\")"="Process: Sync", "State(s) at Back (\"\")"="Exit") -> ("States Out"=w299:string)  [unwired: 12 in]
            n105 = call <vilib>:"Add State(s) to Queue__jki_lib_state_machine.vi"("State(s) in Front (\"\")"="Instrument: Close Hardware", "State(s) in (\"\")"=w304, "State(s) at Back (\"\")"=w299) -> ("States Out"=w303:string)  [unwired: 12 in]
            n106 = call <vilib>:"Add State(s) to Queue__jki_lib_state_machine.vi"("State(s) in Front (\"\")"=w303, "State(s) in (\"\")"=w308) -> ("States Out"=w307:string)  [unwired: 13 in]
          }
          frame "---------- Process ----------" {
            # "Template Separator\n(You can make a copy of, or modify, this frame)"
            n107 = call <vilib>:"Add State(s) to Queue__jki_lib_state_machine.vi"("State(s) in (\"\")"=w313) -> ("States Out"=w312:string)  [unwired: 14 in]
          }
          frame "Process: Sync" {
            n108 = Unbundle By Name(w321) -> ("SMO"=w317:refnum<class "Inst.RP100.lvclass">)
            n109 = call <vilib>:"WaitOnProcessSync.vi"("error in (no error)"=w316, "SMO"=w317) -> ("error out"=w315:errorcluster, "Don't run?"=w320:bool)  [unwired: 7 in, 1 out]
            n110 = Select(t="Data: Cleanup\nEvents: Unregister\nExit", s=w320, f="" ("Empty String Constant")) -> (s? t:f=w314:string)
            n111 = call <vilib>:"Add State(s) to Queue__jki_lib_state_machine.vi"("State(s) in Front (\"\")"=w314, "State(s) in (\"\")"=w324) -> ("States Out"=w323:string)  [unwired: 13 in]
          }
          frame "---------- Events ----------" {
            # "Template Separator\n(You can make a copy of, or modify, this frame)"
            n112 = call <vilib>:"Add State(s) to Queue__jki_lib_state_machine.vi"("State(s) in (\"\")"=w329) -> ("States Out"=w328:string)  [unwired: 14 in]
          }
          frame "Events: Register" {
            n113 = Unbundle By Name(w335) -> ("SMO"=w336:refnum<class "Inst.RP100.lvclass">)
            n114 = call <vilib>:"GetProtectedEvents.vi"("SMO"=w336) -> ("error out"=w334:errorcluster, "SMO Protected Events"=w339:T8, "SMO out"=w333:refnum<class "Inst.RP100.lvclass">)  [unwired: 8 in]
            n115 = call "Inst.RP100.GetPrivateEvents.vi"("Inst.RP100 in"=w333) -> ("error out"=w330:errorcluster, "Inst.RP100 Private Events"=w331:cluster{"MessageToProcess":refnum<user-event>})  [unwired: 8 in, 1 out]
            n116 = register-events(w339, w331) -> (reference out=w340:refnum<event-registration>, error out=w337:errorcluster)  [unwired: 2 in]
            n117 = Merge Errors(w337, w330, w334, w332) -> (w338:errorcluster)
            n118 = call <vilib>:"Add State(s) to Queue__jki_lib_state_machine.vi"("State(s) in (\"\")"=w342) -> ("States Out"=w341:string)  [unwired: 14 in]
          }
          frame "Events: Unregister" {
            n119 = Unregister For Events(event registration refnum=w345, error in=w344) -> (error out=w343:errorcluster)
            n120 = call <vilib>:"Clear Errors.vi"("error in (no error)"=w343) -> ()  [unwired: 5 in, 2 out]
            n121 = call <vilib>:"Add State(s) to Queue__jki_lib_state_machine.vi"("State(s) in (\"\")"=w348) -> ("States Out"=w347:string)  [unwired: 14 in]
          }
          frame "---------- Instrument ----------" {
            n122 = Unbundle By Name(w350) -> ("SMO"=w349:refnum<class "Inst.RP100.lvclass">)
            n123 = Bundle By Name(cluster=w350, "SMO"=w349) -> (w351:T5)
            n124 = call <vilib>:"Add State(s) to Queue__jki_lib_state_machine.vi"("State(s) in (\"\")"=w355) -> ("States Out"=w354:string)  [unwired: 14 in]
          }
          frame "Instrument: Open Hardware" {
            n125 = Unbundle By Name(w360) -> ("SMO"=w359:refnum<class "Inst.RP100.lvclass">)
            n126 = call-dynamic "Open Hardware.vi"("error in (no error)"=w356, "Inst.RP100 in"=w359) -> ("error out"=w357:errorcluster, "Inst.RP100 out"=w358:refnum<class "Inst.RP100.lvclass">)  [unwired: 8 in]
            n127 = Bundle By Name(cluster=w360, "SMO"=w358) -> (w361:T5)
            n128 = call <vilib>:"Add State(s) to Queue__jki_lib_state_machine.vi"("State(s) in (\"\")"=w364) -> ("States Out"=w363:string)  [unwired: 14 in]
          }
          frame "Instrument: Close Hardware" {
            n129 = Unbundle By Name(w369) -> ("SMO"=w368:refnum<class "Inst.RP100.lvclass">)
            n130 = call-dynamic "Close Hardware.vi"("error in (no error)"=w365, "Inst.RP100 in"=w368) -> ("error out"=w366:errorcluster, "Inst.RP100 out"=w367:refnum<class "Inst.RP100.lvclass">)  [unwired: 8 in]
            n131 = Bundle By Name(cluster=w369, "SMO"=w367) -> (w370:T5)
            n132 = call <vilib>:"Add State(s) to Queue__jki_lib_state_machine.vi"("State(s) in (\"\")"=w373) -> ("States Out"=w372:string)  [unwired: 14 in]
          }
          frame "Instrument: setLevel" {
            # "communicate with\nhardware"
            n133 = Unbundle By Name(w379) -> ("SMO"=w377:refnum<class "Inst.RP100.lvclass">, "MessageToProcess.Message.Data"=w374:variant)  [unwired: 1 out]
            n134 = call "Inst.RP100.setLevel.vi"("error in (no error)"=w376, "Variant"=w374, "Inst.RP100 out"=w377) -> ("error out"=w375:errorcluster, "Inst.RP100 out"=w378:refnum<class "Inst.RP100.lvclass">)  [unwired: 7 in]
            n135 = Bundle By Name(cluster=w379, "SMO"=w378) -> (w380:T5)
            n136 = call <vilib>:"Add State(s) to Queue__jki_lib_state_machine.vi"("State(s) in (\"\")"=w383) -> ("States Out"=w382:string)  [unwired: 14 in]
          }
          frame "Instrument: setStrain" {
            # "communicate with\nhardware"
            n137 = Unbundle By Name(w389) -> ("SMO"=w387:refnum<class "Inst.RP100.lvclass">, "MessageToProcess.Message.Data"=w384:variant)  [unwired: 1 out]
            n138 = call "Inst.RP100.setStrain.vi"("error in (no error)"=w386, "data in"=w384, "Inst.RP100 in"=w387) -> ("error out"=w385:errorcluster, "Inst.RP100 out"=w388:refnum<class "Inst.RP100.lvclass">)  [unwired: 7 in]
            n139 = Bundle By Name(cluster=w389, "SMO"=w388) -> (w390:T5)
            n140 = call <vilib>:"Add State(s) to Queue__jki_lib_state_machine.vi"("State(s) in (\"\")"=w393) -> ("States Out"=w392:string)  [unwired: 14 in]
          }
          frame "Instrument: setState" {
            # "communicate with\nhardware"
            n141 = Unbundle By Name(w399) -> ("SMO"=w397:refnum<class "Inst.RP100.lvclass">, "MessageToProcess.Message.Data"=w394:variant)  [unwired: 1 out]
            n142 = call "Inst.RP100.setState.vi"("error in (no error)"=w396, "data in"=w394, "Inst.RP100 in"=w397) -> ("error out"=w395:errorcluster, "Inst.RP100 out"=w398:refnum<class "Inst.RP100.lvclass">)  [unwired: 7 in]
            n143 = Bundle By Name(cluster=w399, "SMO"=w398) -> (w400:T5)
            n144 = call <vilib>:"Add State(s) to Queue__jki_lib_state_machine.vi"("State(s) in (\"\")"=w403) -> ("States Out"=w402:string)  [unwired: 14 in]
          }
          frame "Instrument: getAll" {
            # "communicate with\nhardware"
            n145 = Unbundle By Name(w411) -> ("SMO"=w410:refnum<class "Inst.RP100.lvclass">)  [unwired: 2 out]
            n146 = call "Inst.RP100.getAll.vi"("error in (no error)"=w409, "Inst.RP100 in"=w410) -> ("error out"=w405:errorcluster, "output cluster"=w408:T9, "Inst.RP100 out"=w407:refnum<class "Inst.RP100.lvclass">)  [unwired: 7 in]
            n147 = call <userlib>:"setAllData.vi"("error in (no error)"=w405, "AllData"=w408, "Instrument in"=w407) -> ("error out"=w404:errorcluster, "Instrument out"=w406:refnum<class "Inst.RP100.lvclass">)  [unwired: 7 in]
            n148 = Bundle By Name(cluster=w411, "SMO"=w406) -> (w412:T5)
            n149 = call <vilib>:"Add State(s) to Queue__jki_lib_state_machine.vi"("State(s) in (\"\")"=w415) -> ("States Out"=w414:string)  [unwired: 14 in]
          }
          frame "Instrument: Log" {
            n150 = Unbundle By Name(w424) -> ("SMO"=w417:refnum<class "Inst.RP100.lvclass">)
            n151 = Unbundle By Name(w417) -> ("Data"=w421:T9)
            n152 = call-dynamic "Get SMO Database Paths.vi"("error in (no error)"=w419, "Inst.RP100 in"=w417) -> ("error out"=w420:errorcluster, "Paths"=w423:string, "Inst.RP100 out"=w422:refnum<class "Inst.RP100.lvclass">)  [unwired: 7 in]
            n153 = call <userlib>:"Instrument.logToDatabase.vi"("error in (no error)"=w420, "Data"=w421, "Paths"=w423, "Instrument"=w422) -> ("error out"=w418:errorcluster, "Instrument out"=w416:refnum<class "Inst.RP100.lvclass">)  [unwired: 6 in]
            n154 = Bundle By Name(cluster=w424, "SMO"=w416) -> (w425:T5)
            n155 = call <vilib>:"Add State(s) to Queue__jki_lib_state_machine.vi"("State(s) in (\"\")"=w428) -> ("States Out"=w427:string)  [unwired: 14 in]
          }
          frame "---------- Sequence ----------" {
            n156 = call <vilib>:"Add State(s) to Queue__jki_lib_state_machine.vi"("State(s) in (\"\")"=w433) -> ("States Out"=w432:string)  [unwired: 14 in]
          }
          frame "Sequence: Status" {
            # "Sequence: Status\n(Use this frame to pass the status to the UI, this VI's UI, etc)"
            n157 = call <vilib>:"Add State(s) to Queue__jki_lib_state_machine.vi"("State(s) in (\"\")"=w439) -> ("States Out"=w438:string)  [unwired: 14 in]
            "Status" <- w434
          }
          frame "Sequence: Wait" {
            # "Sequence: Wait\n(Non-Blocking Wait)"
            # "F = repeat this state. wait\nT = go to next state. don't wait"
            n158 = Unbundle By Name(w448) -> ("Running Step"=w441:i32)
            n159 = call <userlib>:"Wait Logic.vi"("error in (no error)"=w444, "Time"=w442) -> ("error out"=w443:errorcluster, "Status String"=w440:string, "Trigger"=w445:bool)  [unwired: 6 in, 1 out]
            n160 = Increment(x=w441) -> (x+1=w455:i32)
            n161 = Select(t=w455, s=w445, f=w441) -> (s? t:f=w446:i32)
            n162 = Select(t=u32 0, s=w445, f=u32 100 ("milliseconds to wait")) -> (s? t:f=w452:u32)
            n163 = call <userlib>:"Wait (ms)__ogtk.vi"("error in (no error)"=w443, "milliseconds to wait"=w452) -> ("error out"=w450:errorcluster)  [unwired: 8 in, 1 out]
            n164 = Bundle By Name(cluster=w448, "Running Step"=w446) -> (w447:T5)
            n165 = call <vilib>:"Build State String with Arguments__JKI_lib_State_Machine.vi"("Arguments (\"\")"=w440, "State"="Sequence: Status") -> ("State with Arguments"=w449:string)  [unwired: 4 in]
            n166 = call <vilib>:"Add State(s) to Queue__jki_lib_state_machine.vi"("State(s) in Front (\"\")"=w449, "State(s) in (\"\")"=w458) -> ("States Out"=w457:string)  [unwired: 13 in]
          }
        }
      }
    }
    frame Error {
    }
  }
  n167 = call-parent "Process.vi"("error in"=w5, "Instrument"=w4) -> ("error out"=w2:errorcluster, "Instrument out"=→"Inst.RP100 out":refnum<class "Inst.RP100.lvclass">)  [unwired: 8 in]
  n168 = Merge Errors(w2, w1) -> (→"error out":errorcluster)
